vi "goToStandby.vi"(8 "error in (no error)":errorcluster, 10 "model in":refnum<class "IModel.lvclass">, 11 "FaultState in":refnum<class "FaultState.lvclass">) -> (0 "error out":errorcluster, 2 "model out":refnum<class "IModel.lvclass">, 3 "FaultState out":refnum<class "FaultState.lvclass">)   [LabVIEW 2016, in "States.lvlib" / "FaultState.lvclass"]
uses:
  FaultState.lvclass
  IModel/IModel.lvclass
  ComponentTemplateCore/ComponentModel/ComponentModel/InternalSignals/clearMessagingError.vi
  ComponentTemplateCore/ComponentModel/ComponentModel/InternalSignals/InternalSignalsGlobals.lvlib
  ComponentTemplateCore/ComponentModel/ComponentModel/InternalSignals/restart.vi
  Typedefs/CommandValue.ctl
  Typedefs/EXATypedefs.lvlib
  ts_sallv_sedspectrometer/DataTypes/logevent_SummaryState.ctl
  ts_sallv_sedspectrometer/SALLV_calibrationSpectrometer.lvlib
  ts_sallv_sedspectrometer/DataTypes/logevent_DetailedState.ctl
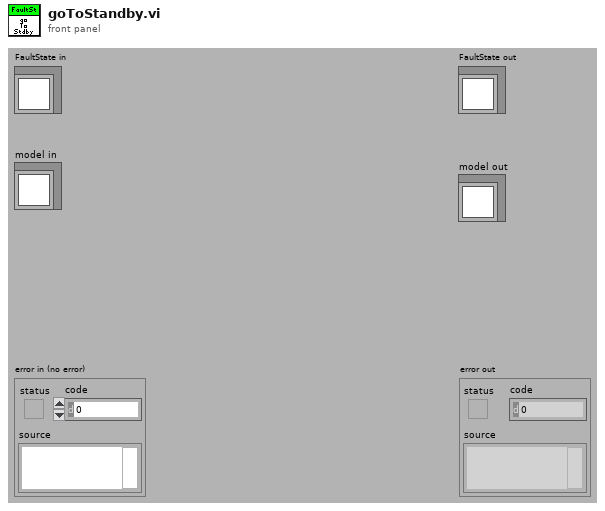
[diagram p1: front panel]
types:
  T1 = typedef "SALLV_calibrationSpectrometer.lvlib/logevent_DetailedState.ctl" = cluster{"detailedState":enum16{"", "DisabledState", "EnabledState", "FaultState", "OfflineState", "StandbyState"}, "priority":i32}
  T2 = typedef "SALLV_calibrationSpectrometer.lvlib/logevent_SummaryState.ctl" = cluster{"summaryState":enum16{"", "DisabledState", "EnabledState", "FaultState", "OfflineState", "StandbyState"}, "priority":i32}
  T3 = typedef "EXATypedefs.lvlib/CommandValue.ctl" = enum16{"Disable", "Enable", "Exit", "GoToStandby", "OnHeartbeat", "OnIncomingMessagingError", "OnInterrupt", "Start", "CaptureSpectImage", "SetSpectTempSetpoint", "StopImageCapture"}
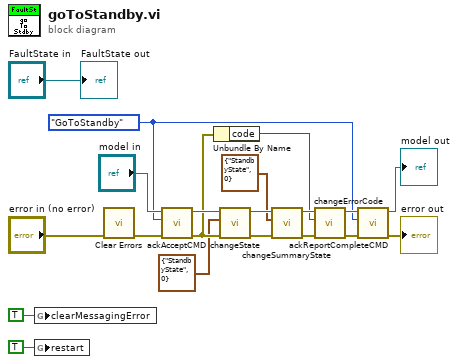
[diagram p0: block diagram]
diagram:
  w3 = CommandValue."GoToStandby" ("CommandValue")
  n1 = global write "clearMessagingError.vi" "clearMessagingError"(TRUE ("clearMessagingError")) -> ()
  n2 = global write "restart.vi" "restart"(TRUE ("restart")) -> ()
  n3 = call <vilib>:"Clear Errors.vi"("error in (no error)"="error in (no error)") -> ("error out"=w11:errorcluster)  [unwired: 5 in, 1 out]
  n4 = call-dynamic "ackAcceptCMD.vi"("error in (no error)"=w11, "CommandValue"=w3, "IModel in"="model in") -> ("error out"=w8:errorcluster, "IModel out"=w9:refnum<class "IModel.lvclass">)  [unwired: 7 in]
  n5 = Unbundle By Name(w8) -> ("code"=w16:i32)
  n6 = call-dynamic "changeState.vi"("error in (no error)"=w8, "DetailedState"=T1 {"detailedState"=enum."StandbyState", "priority"=0} ("logevent_DetailedState"), "IModel in"=w9) -> ("error out"=w18:errorcluster, "IModel out"=w19:refnum<class "IModel.lvclass">)  [unwired: 7 in]
  n7 = call-dynamic "changeSummaryState.vi"("error in (no error)"=w18, "logevent_SummaryState"=T2 {"summaryState"=enum."StandbyState", "priority"=0}, "IModel in"=w19) -> ("error out"=w15:errorcluster, "IModel out"=w17:refnum<class "IModel.lvclass">)  [unwired: 7 in]
  n8 = call-dynamic "changeErrorCode.vi"("error in (no error)"=w15, "error.code"=w16, "IModel in"=w17) -> ("error out"=w7:errorcluster, "IModel out"=w4:refnum<class "IModel.lvclass">)  [unwired: 7 in]
  n9 = call-dynamic "ackReportCompleteCMD.vi"("error in (no error)"=w7, "CommandValue"=w3, "IModel in"=w4) -> ("error out"=→"error out":errorcluster, "IModel out"=→"model out":refnum<class "IModel.lvclass">)  [unwired: 7 in]
  "FaultState out" <- "FaultState in"
